vi "write_pulse_count.vi"(10 "Address":u8, 11 "Pulse count":i16) -> ()   [LabVIEW 2012]
uses:
  Common/i2c_command.ctl
  <vilib>/rvi/DataTransferAndStorage/Container/Common/niFpgaContainerExecOnDevCompGetState.vi
  <vilib>/rvi/Emulation/niFpgaSctlEmulationGetInTimedLoop.vi
  <vilib>/rvi/DataTransferAndStorage/Container/Common/niFpgaContainerGetUniqueNameForEmu.vi
  <vilib>/rvi/FIFO/Fifo_Resource/nirvififoEmulationSetSize.vi
  <vilib>/rvi/errors/niFpgaSetErrorForExecOnDevCompSimple.vi
  <vilib>/rvi/eio/common/nirviEmuReportErrorAndStop.vi
  <vilib>/rvi/Emulation/niFpgaSctlEmulationFifoFullMgr.vi
  <vilib>/rvi/Emulation/niFpgaSctlEmulationResourceMgr.vi
  <vilib>/rvi/interface/RandomDataEmulation/nirviRandomDataFPGAFIFO.vi
  <vilib>/rvi/interface/RandomDataEmulation/niFpgaRandomDataHandleErrors.vi
  <vilib>/rvi/DataTransferAndStorage/Container/XNode/niFpgaContainer.xnode
  <vilib>/rvi/FIFO/Fifo_Resource/niFpgaFifoEmulationRefIn.vi
panel:
  # "Motor command, signed 12 bit"
  # "I2C address, U8."
  # "Write FIFO for bus controller."
  # "Write the NSD2101 pulse count register."
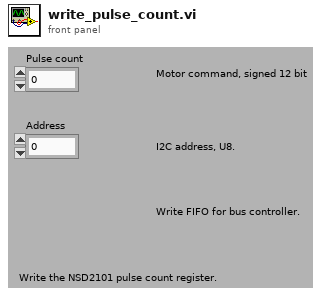
[diagram p1: front panel]
types:
  T1 = typedef "i2c_command.ctl" = enum8{"invalid", "start_write", "start_read", "stop", "sequence"}
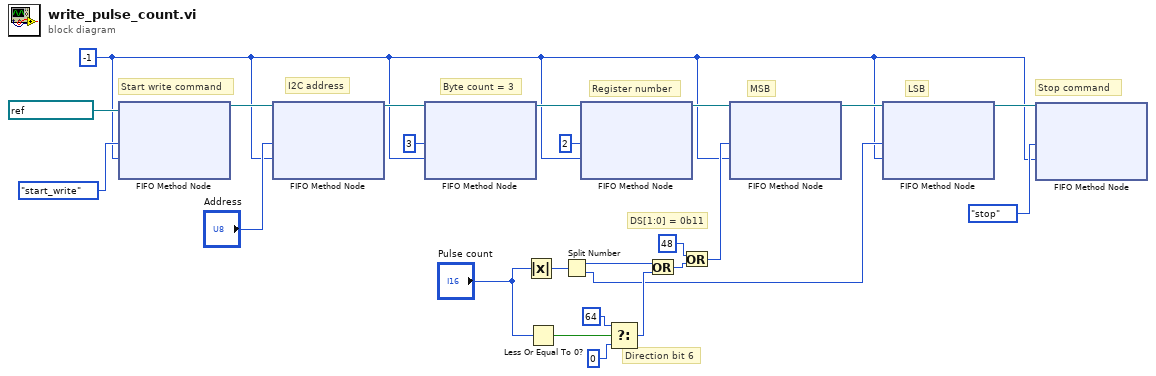
[diagram p0: block diagram]
diagram:
  w1 = -1 ("Timeout")
  # "Stop command"
  # "Byte count = 3"
  # "I2C address"
  # "Start write command"
  # "LSB"
  # "MSB"
  # "Register number"
  # "DS[1:0] = 0b11"
  # "Direction bit 6"
  n1 = xnode ("FIFO Method Node")("Element"=i2c_command."start_write" ("Command"), "Timeout"=w1, "FIFO In"=refnum<k21> "Local write" ("FIFO")) -> ("FIFO Out"=w9:refnum<k21>)  [unwired: 1 out]
  n2 = xnode ("FIFO Method Node")("Element"="Address", "Timeout"=w1, "FIFO In"=w9) -> ("FIFO Out"=w6:refnum<k21>)  [unwired: 1 out]
  n3 = xnode ("FIFO Method Node")("Element"=u8 3, "Timeout"=w1, "FIFO In"=w6) -> ("FIFO Out"=w5:refnum<k21>)  [unwired: 1 out]
  n4 = Absolute Value(x="Pulse count") -> (abs(x)=w24:i16)
  n5 = Less Or Equal To 0?(x="Pulse count") -> (x <= 0?=w19:bool)
  n6 = Split Number(x=w24) -> (hi(x)=w17:u8, lo(x)=w11:u8)
  n7 = xnode ("FIFO Method Node")("Element"=u8 2 ("lo(x)"), "Timeout"=w1, "FIFO In"=w5) -> ("FIFO Out"=w14:refnum<k21>)  [unwired: 1 out]
  n8 = Select(t=u8 64 ("lo(x)"), s=w19, f=u8 0 ("lo(x)")) -> (s? t:f=w18:u8)
  n9 = Or(x=w17, y=w18) -> (x .or. y?=w16:u8)
  n10 = Or(x=u8 48 ("lo(x)"), y=w16) -> (x .or. y?=w12:u8)
  n11 = xnode ("FIFO Method Node")("Element"=w12, "Timeout"=w1, "FIFO In"=w14) -> ("FIFO Out"=w13:refnum<k21>)  [unwired: 1 out]
  n12 = xnode ("FIFO Method Node")("Element"=w11, "Timeout"=w1, "FIFO In"=w13) -> ("FIFO Out"=w3:refnum<k21>)  [unwired: 1 out]
  n13 = xnode ("FIFO Method Node")("Element"=i2c_command."stop" ("Command"), "Timeout"=w1, "FIFO In"=w3) -> ()  [unwired: 2 out]
